vi "Create Recorder File Path.vi"(11 "T: Move_Shoot\nF: Shoot_Move":bool) -> (3 "Path":path)   [LabVIEW 2011]
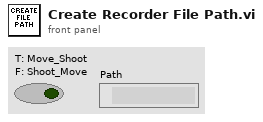
[diagram p1: front panel]
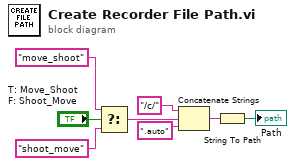
[diagram p0: block diagram]
diagram:
  n1 = Select(t="move_shoot", s="T: Move_Shoot\nF: Shoot_Move", f="shoot_move") -> (s? t:f=w2:string)
  n2 = Concatenate Strings("/c/", w2, ".auto") -> (w1:string)
  n3 = String To Path(string=w1) -> (path=→"Path":path)
